vi "State_Exit.vi"(8 "error in (no error)":errorcluster, 9 "Parameter":variant, 10 "Command":string, 11 "launcher in":refnum<class "launcher.lvclass">) -> (0 "error out":errorcluster, 2 "Debug Message":string, 3 "launcher out":refnum<class "launcher.lvclass">, 4 "Stop?":bool)   [LabVIEW 2021, in "launcher.lvclass"]
uses:
  launcher.lvclass
  C:/Program Files (x86)/National Instruments/LabVIEW 2021/user.lib/S2 Labs/Module Framework/Modules/Base/Module.lvclass
  <userlib>/S2 Labs/Queued State Machine/TypeDefs/Queue Message.ctl
  <userlib>/S2 Labs/Queued State Machine/TypeDefs/States.ctl
  <userlib>/S2 Labs/Module Framework/Modules/Base/Module.lvclass/Module.ctl
  <userlib>/S2 Labs/Queued State Machine/QSM.lvclass/QSM.ctl
  e13ef6b2-5e2c-44f9-85ad-fd9b0373f98f.vi
  <userlib>/S2 Labs/Module Framework/Modules/Base/Read Caller Queue.vi
  <userlib>/S2 Labs/Module Framework/Modules/Base/Read Logging Queue.vi
  <userlib>/S2 Labs/Queued State Machine/Enqueue Element.vi
  <userlib>/S2 Labs/Queued State Machine/Callback Notifier/Obtain Callback Notifier.vi
  <userlib>/S2 Labs/Queued State Machine/Callback Notifier/Release Reply Notifier.vi
  <userlib>/S2 Labs/Queued State Machine/QSM.lvclass
  <userlib>/S2 Labs/Queued State Machine/Callback Notifier/Callback Notifier.lvclass
  <userlib>/S2 Labs/Module Framework/Modules/Base/Module.lvclass
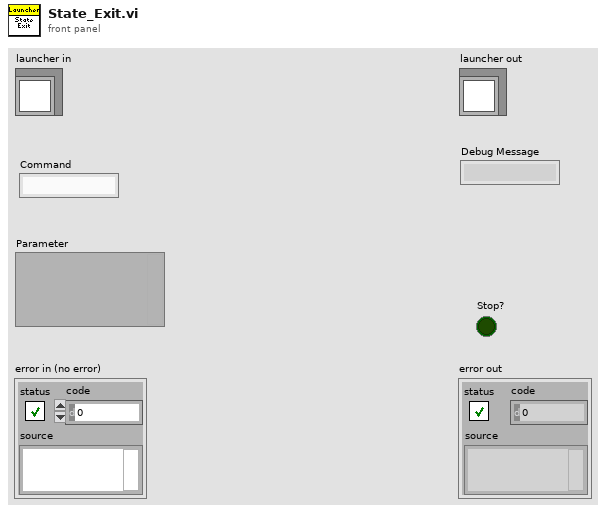
[diagram p1: front panel]
types:
  T1 = typedef "QSM.lvclass/Queue Message.ctl" = cluster{"State":T2, "Command":string, "Parameter":variant}
  T2 = typedef "QSM.lvclass/States.ctl" = enum16{"Waiting", "Init", "ExecCMD", "Read Config", "Write Config", "Launch", "Connect", "Recovery", "Clean Up", "Exit"}
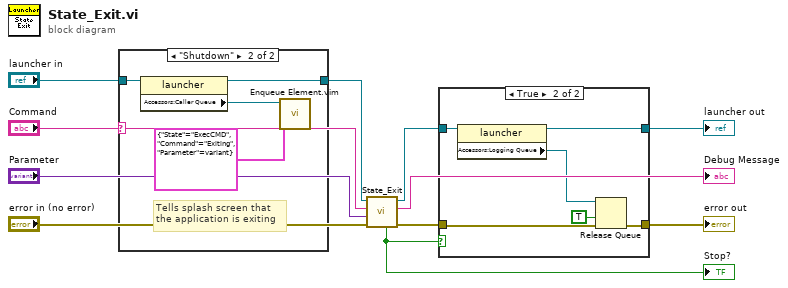
[diagram p0: block diagram]
diagram:
  n1 = case shown="\"Shutdown\"" "Command" {
    tunnel: "launcher in" -> [w12 w15]
    tunnel: [w12 w16] -> w2
    frame Default {
    }
    frame "Shutdown" {
      # "Tells splash screen that\nthe application is exiting"
      n2 = property class="launcher"(reference=w15) -> (reference out=w16:refnum<class "launcher.lvclass">, "Accessors:Caller Queue"=w14:refnum<class "QSM.lvclass">)  [unwired: 1 in, 1 out]
      n3 = call "Enqueue Element.vim"("Message"=T1 {"State"=enum."ExecCMD", "Command"="Exiting", "Parameter"=variant}, "QSM in"=w14) -> ()  [unwired: 5 in, 5 out]
    }
  }
  n4 = call-parent "State_Exit.vi"("error in (no error)"="error in (no error)", "Parameter"="Parameter", "Command"="Command", "Module in"=w2) -> ("error out"=w7:errorcluster, "Debug Message"=→"Debug Message":string, "Module out"=w5:refnum<class "launcher.lvclass">, "Stop?"=w6:bool)  [unwired: 4 in]
  "Stop?" <- w6
  n5 = case shown="True" w6 {
    tunnel: [w17 w21] -> w8
    tunnel: w7 -> [w17 w22]
    tunnel: w5 -> [w18 w23]
    tunnel: [w18 w24] -> w4
    frame False {
    }
    frame True {
      n6 = property class="launcher"(reference=w23) -> (reference out=w24:refnum<class "launcher.lvclass">, "Accessors:Logging Queue"=w20:refnum<queue>)  [unwired: 1 in, 1 out]
      n7 = Release Queue(queue=w20, force destroy? (F)=TRUE, error in (no error)=w22) -> (error out=w21:errorcluster)  [unwired: 2 out]
    }
  }
  "error out" <- w8
  "launcher out" <- w4
